vi "MultiAxisControl.vi"() -> ()   [LabVIEW 2010]
uses:
  Utility/AxisControl.ctl
  Motion/AbortSingle.vi
  Motion/MoveIncSingle.vi
  Motion/FreerunSingle.vi
  Motion/EnableSingle.vi
  Motion/DisableSingle.vi
  Motion/FaultAckSingle.vi
  Motion/HomeSingle.vi
  Parameters/GetAxisParameterString.vi
  Parameters/GetAxisParameterDouble.vi
panel:
  out "Status":string
  in  "StopProgram":bool caption="Stop"
  out "do stop":bool
  in  "stop":bool
  out "Error":string
  in  "Init":bool=TRUE
  in  "Abort Motion":bool
  in  "Reset Controller":bool
  in  "In Task:":i32(ring)=1 items=["Auxiliary", "T1", "T2", "T3", "T4"]
  in  "ExecuteProgram":bool caption="Execute"
  in  "Program:":path
  in  "Axes":T1[](array[typedef])
  in  "Status":string
  in  "Execute":bool
  in  "Command:":string
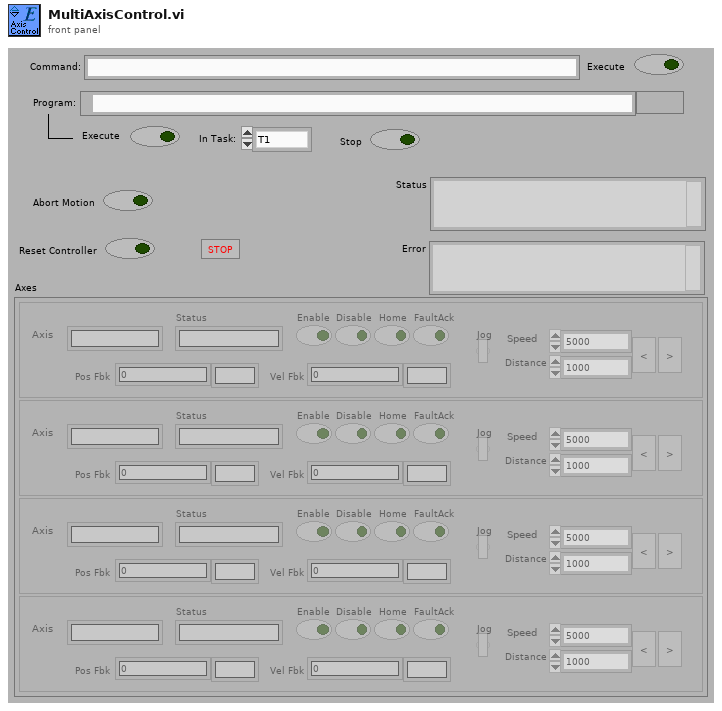
[diagram p1: front panel]
types:
  T1 = typedef "AxisControl.ctl" = cluster{"Axis":string, "Enable":bool, "Disable":bool, "Home":bool, "FaultAck":bool, "Jog":bool, "Speed":dbl, "Distance":dbl, "Jog Left":bool, "Jog Right":bool, "Status":string, "Pos Fbk":dbl, "Vel Fbk":dbl, "Pos Units":string, "Vel Units":string}
  T2 = cluster{"new reference":refnum<k24>, "Event Callback":refnum<k27>, "ControllerDiagPacket":refnum<user-event>, "Event Registration Refnum":refnum<event-registration>}
  T3 = enum32{"invalid app kind", "Development System", "Run Time System", "Student Edition", "Embedded LabVIEW", "Evaluation", "Custom"}
  T4 = cluster{"Axis":string, "Enable":bool, "Disable":bool, "Home":bool, "FaultAck":bool, "Jog":bool, "Speed":dbl, "Distance":dbl, "Jog Left":bool, "Jog Right":bool, "Status":string, "Pos Fbk":dbl, "Vel Fbk":dbl, "Pos Units":string, "Vel Units":string}
  T5 = typedef "AxisDiagPacket.ctl" = cluster{"Axis Name":string, "Acceleration Command":dbl, "Amplifier Temperature":sgl, "Analog Input 0":dbl, "Analog Input 1":dbl, "Analog Output 0":dbl, "Analog Output 1":dbl, "Axis Fault (num)":i32, "Axis Fault (str)":string, "Axis Fault (bits)":cluster{"AmplifierFault":bool, "AmplifierTemperatureFault":bool, "CcwEndOfTravelLimitFault":bool, "CcwSoftwareLimitFault":bool, "CommunicationLostFault":bool, "CwEndOfTravelLimitFault":bool, "CwSoftwareLimitFault":bool, "EmergencyStopFault":bool, "EncoderFault":bool, "ExternalFault":bool, "FeedbackScalingFault":bool, "HallSensorFault":bool, "MarkerSearchFault":bool, "MaxVelocityCommandFault":bool, "MotorTemperatureFault":bool, "None":bool, "OverCurrentFault":bool, "PositionErrorFault":bool, "PositionFeedbackFault":bool, "VelocityErrorFault":bool, "VelocityFeedbackFault":bool, "VoltageClampFault":bool, "PowerSupplyFault":bool}, "Axis Status (num)":i32, "Axis Status (str)":string, "Axis Status (bits)":cluster{"AccelerationPhase":bool, "AutofocusActive":bool, "BrakeOutput":bool, "CalibrationActive":bool, "CalibrationEnabled":bool, "CcwEndOfTravelLimitInput":bool, "CommandShapingFilterDone":bool, "CosineEncoderError":bool, "CurrentClamp":bool, "CwEndOfTravelLimitInput":bool, "DecelerationPhase":bool, "EmergencyStopInput":bool, "Enabled":bool, "GantryMasterActive":bool, "GantryModeActive":bool, "HallAInput":bool, "HallBInput":bool, "HallCInput":bool, "Homed":bool, "HomeLimitInput":bool, "Homing":bool, "InPosition":bool, "InPosition2":bool, "JoystickControl":bool, "MarkerInput":bool, "MasterMotionSuppressed":bool, "MasterSlaveControl":bool, "MotionIsCw":bool, "MoveActive":bool, "None":bool, "PositionCaptureActive":bool, "ServoControl":bool, "SineEncoderError":bool}, "Current Command":sgl, "Current Error":sgl, "Current Feedback":sgl, "Digital Input 0":i32, "Digital Input 1":i32, "Digital Input 2":i32, "Digital Output 0":i32, "Digital Output 1":i32, "Digital Output 2":i32, "Position Feedback Auxiliary":dbl, "Position Command":dbl, "Position Error":dbl, "Position Feedback":dbl, "Program Position Command":dbl, "Program Position Error":dbl, "Program Position Feedback":dbl, "Velocity Command":dbl, "Velocity Error":dbl, "Velocity Feedback":dbl}
  T6 = cluster{"Axis":string, "Enable":bool, "Disable":bool, "Home":bool, "FaultAck":bool, "Jog":bool, "Speed":dbl, "Distance":dbl, "Jog Left":bool, "Jog Right":bool, "Status":string, "Pos Fbk":dbl, "Vel Fbk":dbl, "Pos Units":string, "Vel Units":string}[]
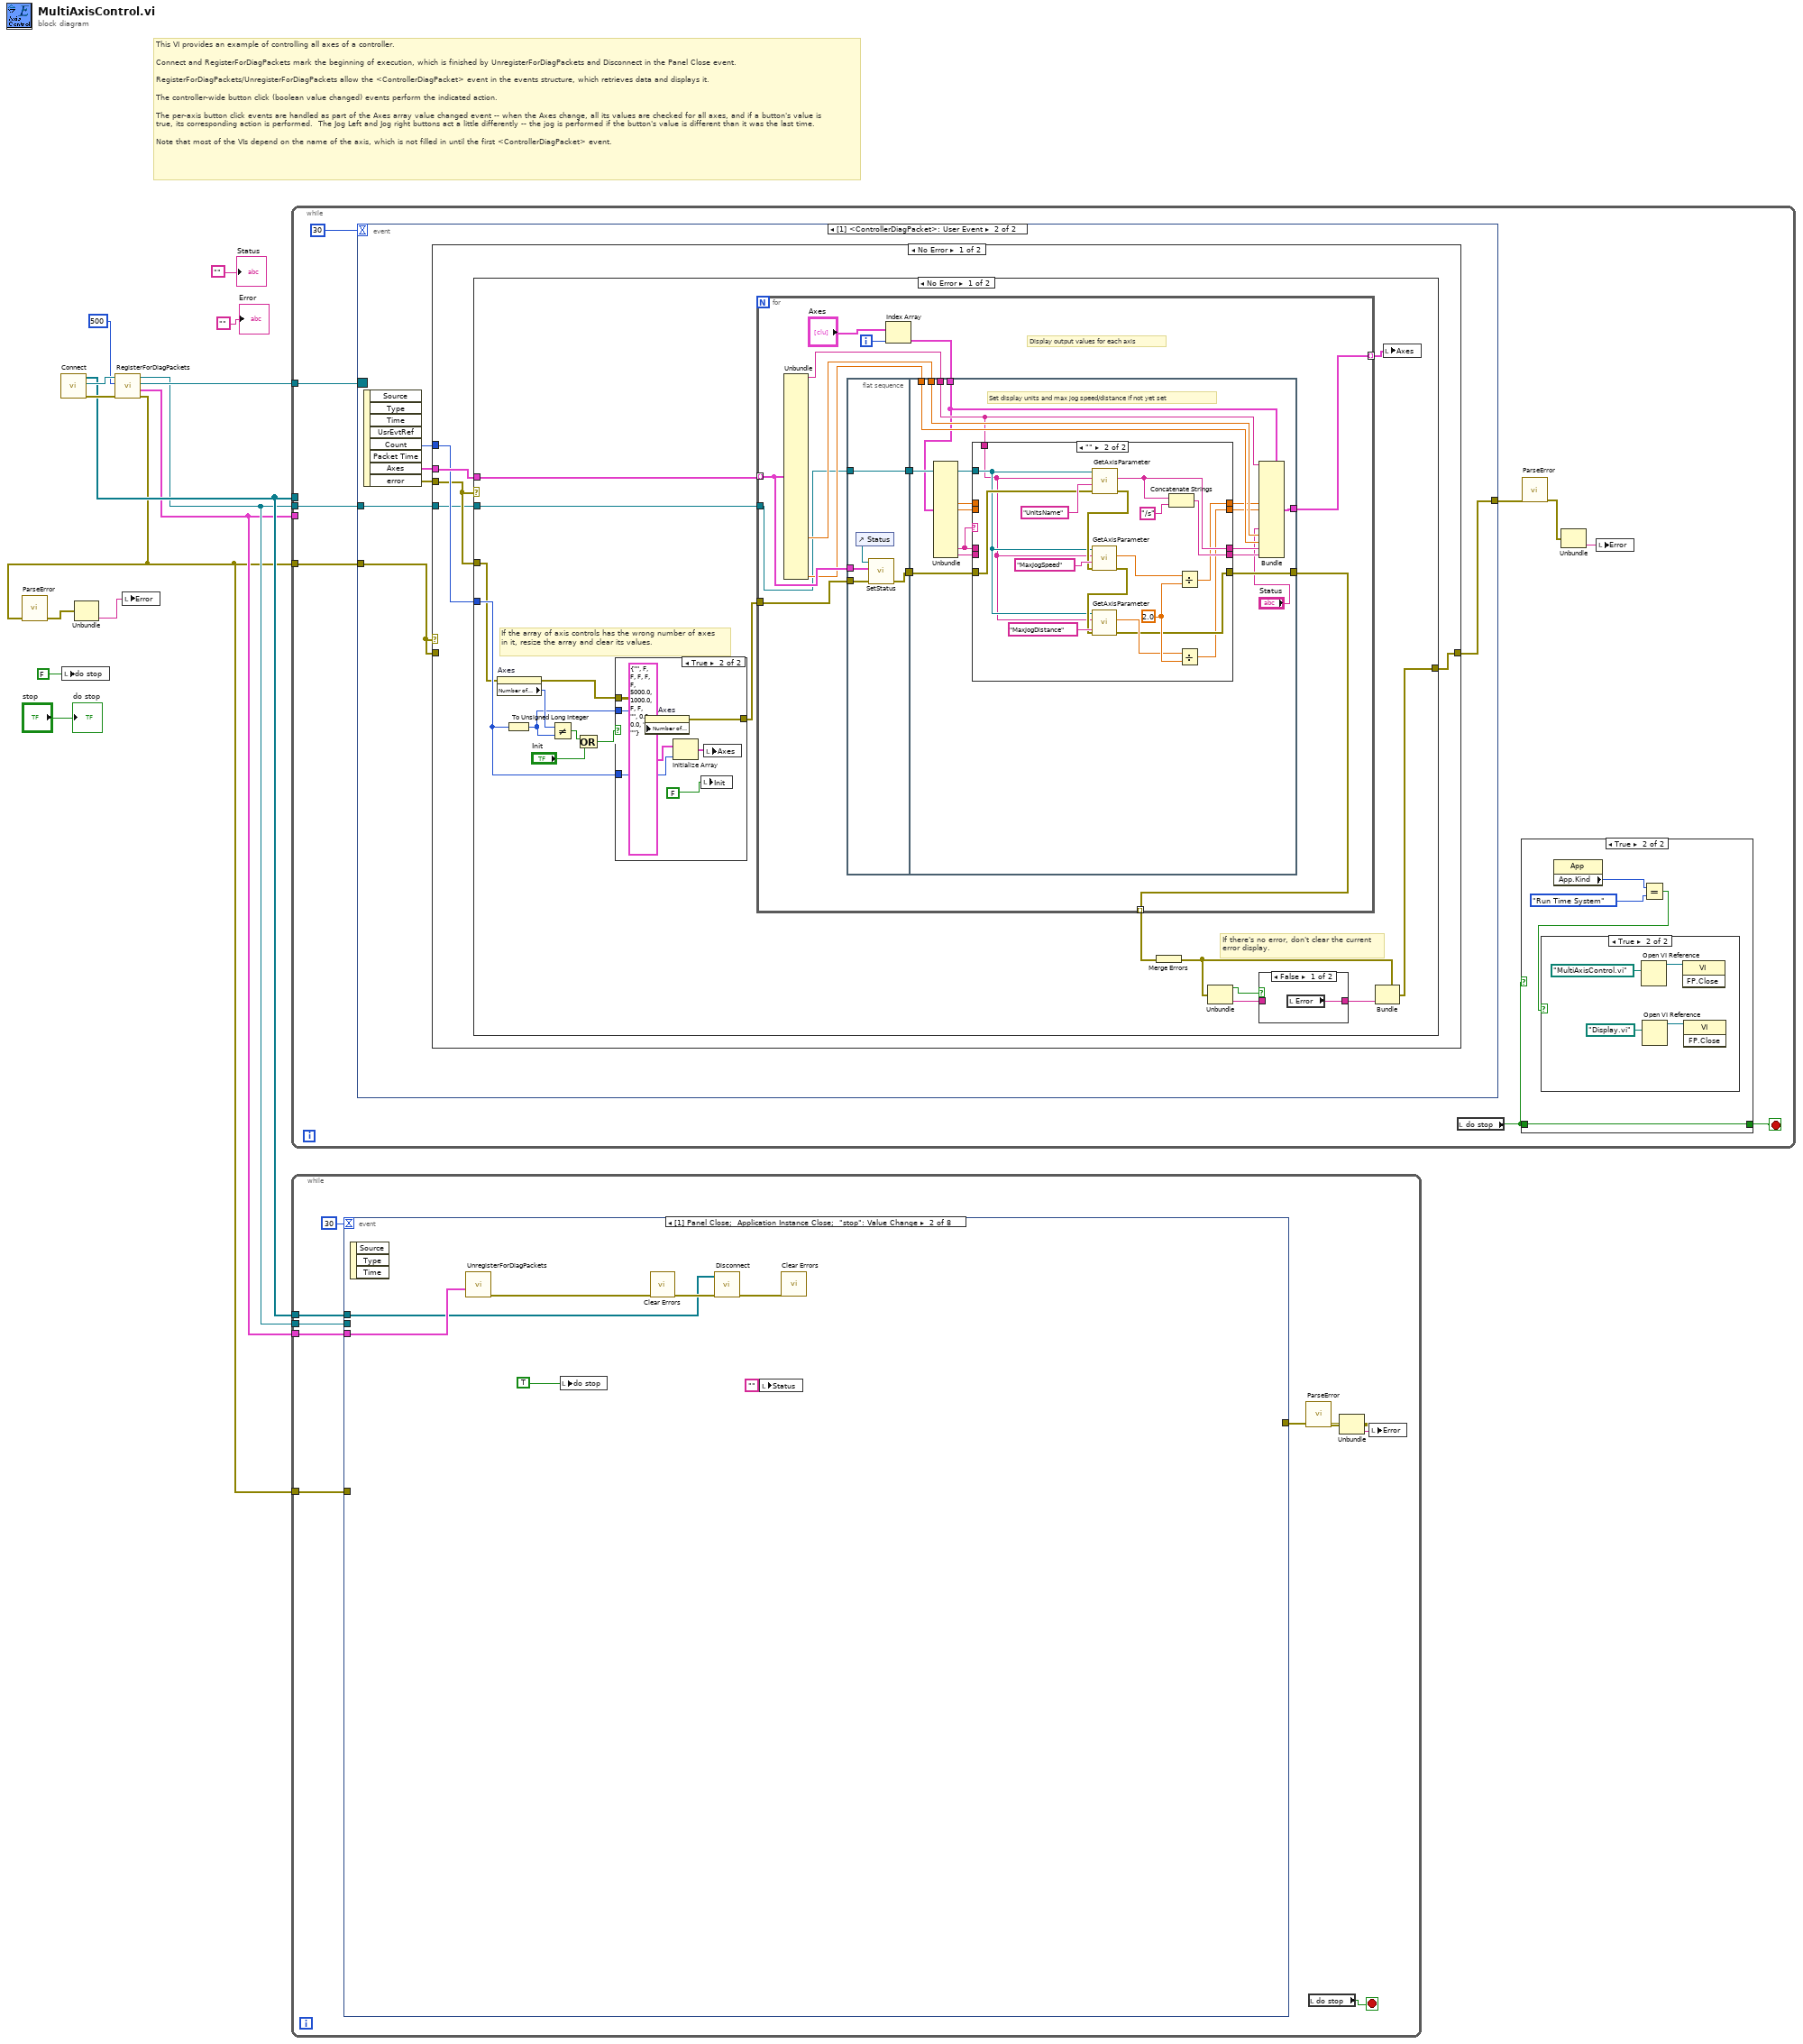
[diagram p0: block diagram]
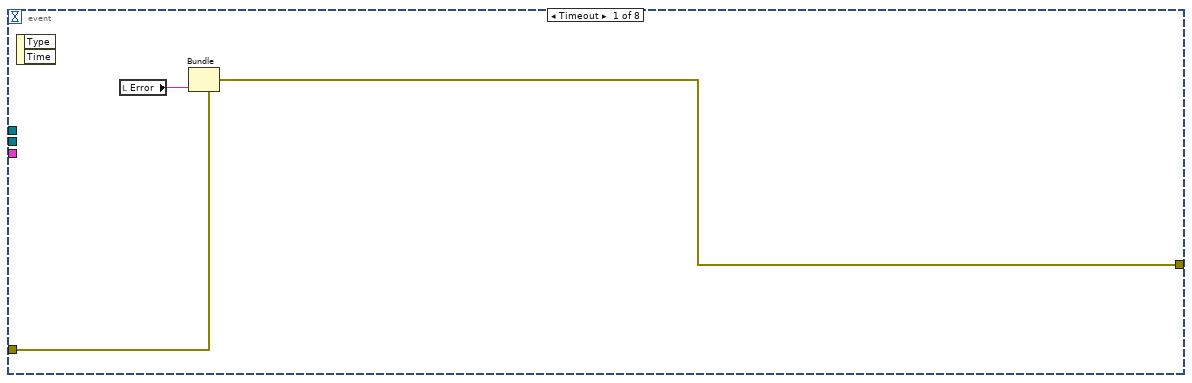
[diagram p2: hidden frame]
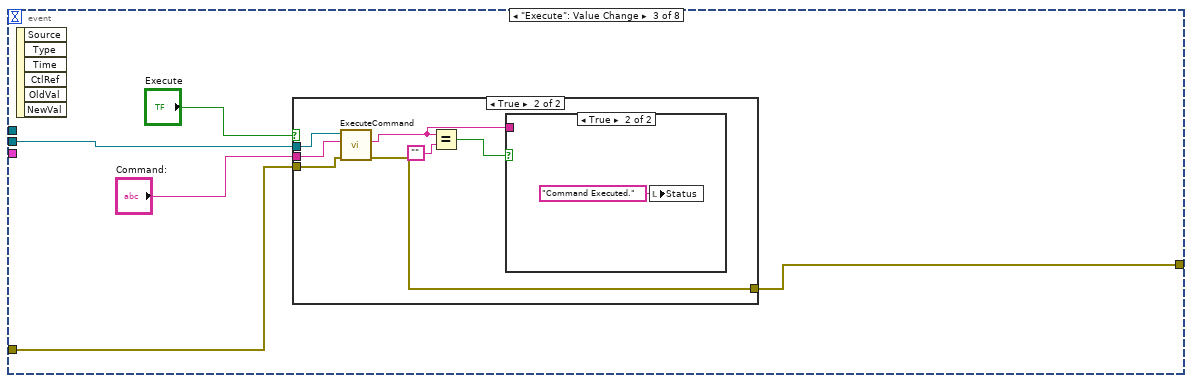
[diagram p3: hidden frame]
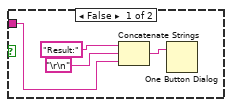
[diagram p5: hidden frame]
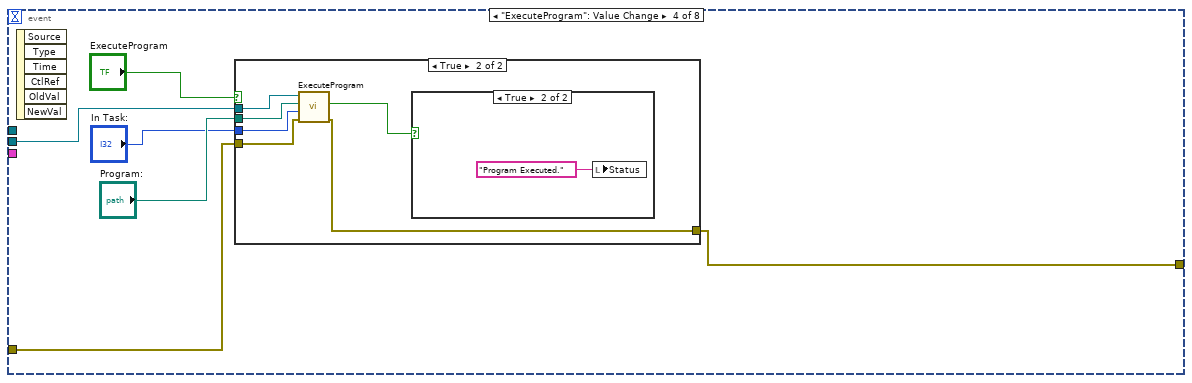
[diagram p6: hidden frame]
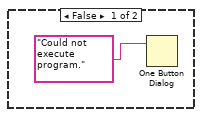
[diagram p8: hidden frame]
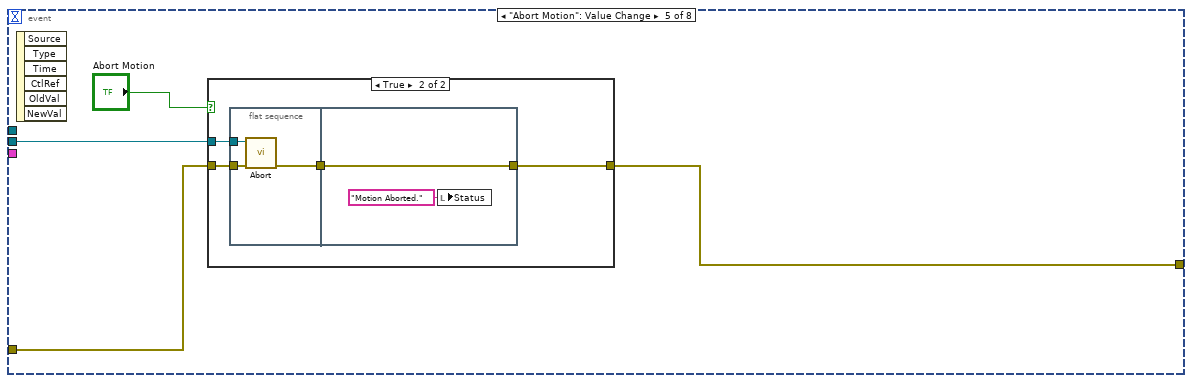
[diagram p9: hidden frame]
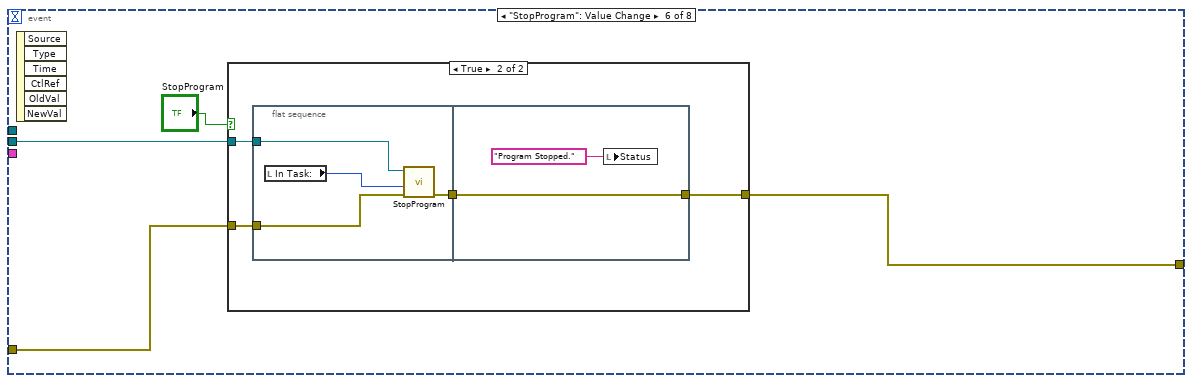
[diagram p11: hidden frame]
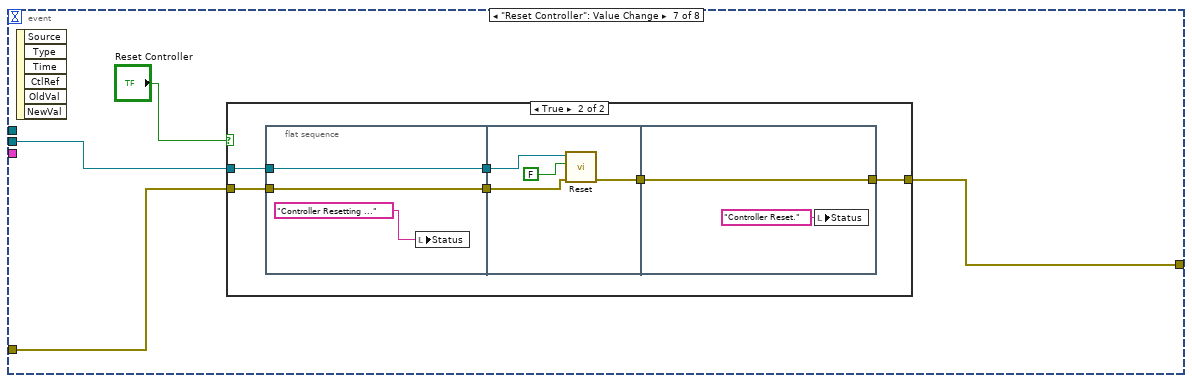
[diagram p13: hidden frame]
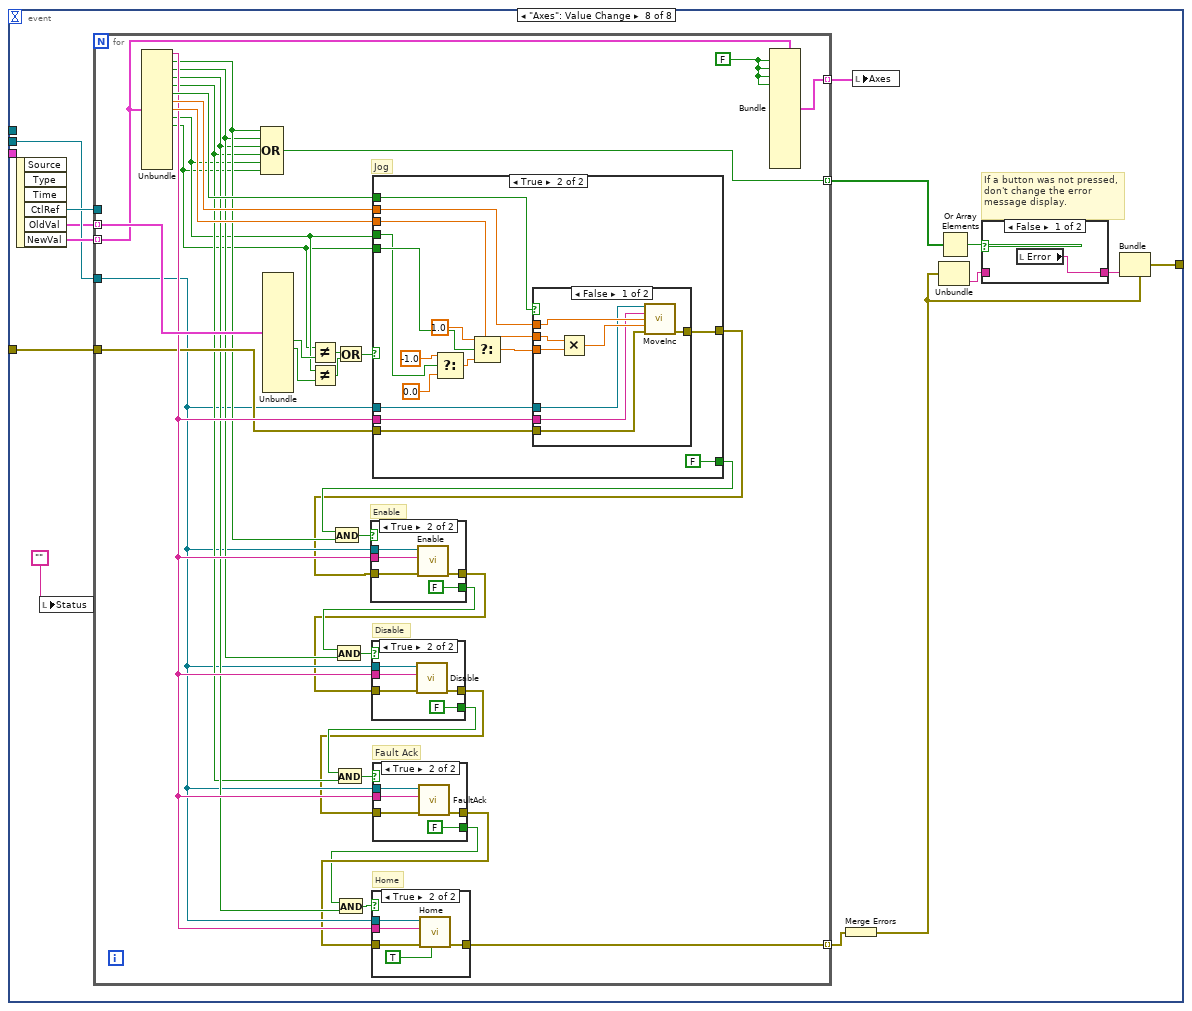
[diagram p15: hidden frame]
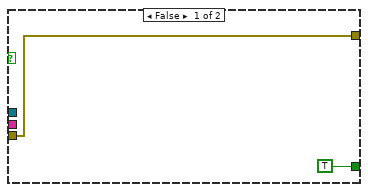
[diagram p17: hidden frame]
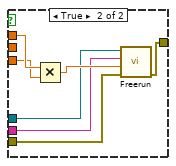
[diagram p18: hidden frame]
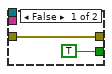
[diagram p19: hidden frame]
diagram:
  # "This VI provides an example of controlling all axes of a controller. \n\nConnect and RegisterForDiagPackets mark the beginning of execution, which is finished by UnregisterForDiagPackets and Disconnect in the Panel Close event.\n\nRegisterForDiagPackets/UnregisterForDiagPackets allow the <ControllerDiagPacket> event in the events structure, which retrieves data and displays it.\n\nThe controller-wide button click (boolean value changed) events perform the indicated action.\n\nThe per-axis button click events are handled as part of the Axes array value changed event -- when the Axes change, all its values are checked for all axes, and if a button's value is true, its corresponding action is performed.  The Jog Left and Jog right buttons act a little differently -- the jog is performed if the button's value is different than it was the last time.\n\nNote that most of the VIs depend on the name of the axis, which is not filled in until the first <ControllerDiagPacket> event."
  n1 = call "Connect.vi"() -> ("error out"=w12:errorcluster, "controller"=w13:refnum<k24>, "controllers"=w7:refnum<k24>[])  [unwired: 9 in]
  n2 = local write "do stop"(FALSE ("do stop")) -> ()
  n3 = call "RegisterForDiagPackets.vi"("error in (no error)"=w12, "refresh interval (default)"=500, "Controller in"=w13) -> ("error out"=w4:errorcluster, "Even Metadata"=w5:T2, "Event Registration Refnum"=w14:refnum<event-registration>, "Controller out"=w6:refnum<k24>)  [unwired: 4 in]
  n4 = call "ParseError.vi"("error in (no error)"=w4) -> ("error out"=w9:errorcluster)  [unwired: 10 in]
  n5 = Unbundle(w9) -> ("source"=w10:string)  [unwired: 2 out]
  n6 = local write "Error"(w10) -> ()
  n7 = while {
    tunnel: w14 -> [w20]
    tunnel: w5 -> [_]
    tunnel: w6 -> [w18]
    tunnel: w7 -> [_]
    tunnel: w4 -> [w17]
    stop <- w16 stop-if-true
    n8 = event shown="[1] <ControllerDiagPacket>: User Event" {
      selector: w20 -> [_ _]
      dyn-events: _ -> [_ _]
      timeout: 30 -> [_ _]
      tunnel: [w33 w41] -> w19
      tunnel: w18 -> [_ w40]
      tunnel: w17 -> [w35 w39]
      event Timeout {
        n9 = event-data() -> ()  [unwired: 1 in, 2 out]
        n10 = local read "Error"() -> (w34:string)
        n11 = Bundle(cluster=w35, "source"=w34) -> (w33:errorcluster)  [unwired: 2 in]
      }
      event User Event {
        n12 = event-data() -> ("Count"=w38:i32, "Axes"=w37:T5[], "error"=w36:errorcluster)  [unwired: 1 in, 5 out]
        n13 = case shown="No Error" w39 {
          tunnel: w37 -> [w46 _]
          tunnel: [w45 w133] -> w41
          tunnel: w38 -> [w44 _]
          tunnel: w36 -> [w43 _]
          tunnel: w39 -> [_ w133]
          tunnel: w40 -> [w42 _]
          frame No Error {
            n14 = case shown="No Error" w43 {
              tunnel: w46 -> [w64 _]
              tunnel: [w53 w132] -> w45
              tunnel: w43 -> [w49 w132]
              tunnel: w44 -> [w58 _]
              tunnel: w42 -> [w47 _]
              frame No Error {
                # "If there's no error, don't clear the current error display."
                # "If the array of axis controls has the wrong number of axes in it, resize the array and clear its values."
                n15 = property on="Axes" class="Arr (strict)"(error in=w49) -> (error out=w48:errorcluster, "Number of Rows"=w60:u32)  [unwired: 1 in, 1 out]
                n16 = To Unsigned Long Integer(number=w58) -> (unsigned 32bit integer=w59:u32)
                n17 = Not Equal?(x=w60, y=w59) -> (x != y?=w57:bool)
                n18 = Or(x=w57, y="Init") -> (x .or. y?=w56:bool)
                n19 = case shown="True" w56 {
                  tunnel: w48 -> [w124 w131]
                  tunnel: [w124 w130] -> w63
                  tunnel: w59 -> [_ w126]
                  tunnel: w58 -> [_ w127]
                  frame False {
                  }
                  frame True {
                    n20 = property on="Axes" class="Arr (strict)"(error in=w131, "Number of Rows"=w126) -> (error out=w130:errorcluster)  [unwired: 1 in, 1 out]
                    n21 = Initialize Array(T4 {"Axis"="", "Enable"=FALSE, "Disable"=FALSE, "Home"=FALSE, "FaultAck"=FALSE, "Jog"=FALSE, "Speed"=5000.0, "Distance"=1000.0, "Jog Left"=FALSE, "Jog Right"=FALSE, "Status"="", "Pos Fbk"=0.0, "Vel Fbk"=0.0, "Pos Units"="", "Vel Units"=""} ("Axis"), w127) -> (w129:T6)
                    n22 = local write "Init"(FALSE ("Init")) -> ()
                    n23 = local write "Axes"(w129) -> ()
                  }
                }
                n24 = for {
                  tunnel: w63 -> [w78]
                  tunnel: w64 -> [w79] mode=indexing
                  tunnel: [w77] -> w62 mode=indexing
                  tunnel: [w70] -> w61 mode=indexing
                  tunnel: w47 -> [w68]
                  i -> [w73]
                  # "Display output values for each axis"
                  n25 = Unbundle(w79) -> ("Axis Name"=w76:string, "Position Feedback"=w72:dbl, "Velocity Feedback"=w71:dbl)  [unwired: 29 out]
                  n26 = flat-sequence {
                    tunnel: w79 -> [w83]
                    tunnel: w78 -> [w82]
                    tunnel: [w81] -> w69
                    tunnel: w68 -> [w80]
                    tunnel: [w80] -> w67
                    tunnel: w74 -> [w94]
                    tunnel: w76 -> [w96]
                    tunnel: w72 -> [w100]
                    tunnel: w71 -> [w99]
                    tunnel: w69 -> [w97]
                    tunnel: w67 -> [w95]
                    tunnel: [w101] -> w77
                    tunnel: [w98] -> w70
                    frame #0 {
                      n27 = control-ref of="Status"() -> (w84:refnum<vi>)
                      n28 = call "SetStatus.vi"("error in (no error)"=w82, "AxisDiagPacket"=w83, "Status string"=w84) -> ("error out"=w81:errorcluster)  [unwired: 8 in]
                    }
                    frame #1 {
                      # "Set display units and max jog speed/distance if not yet set"
                      n29 = Unbundle(w94) -> ("Speed"=w89:dbl, "Distance"=w88:dbl, "Pos Units"=w93:string, "Vel Units"=w92:string)  [unwired: 11 out]
                      n30 = case shown="\"\"" w93 {
                        tunnel: w95 -> [_ w108]
                        tunnel: [w106 w111] -> w98
                        tunnel: w97 -> [w106 w121]
                        tunnel: w96 -> [_ w107]
                        tunnel: w93 -> [w104 _]
                        tunnel: w92 -> [w105 _]
                        tunnel: [w105 w120] -> w91
                        tunnel: [w104 w119] -> w90
                        tunnel: w89 -> [w103 _]
                        tunnel: w88 -> [w102 _]
                        tunnel: [w103 w110] -> w87
                        tunnel: [w102 w109] -> w86
                        frame Default {
                        }
                        frame "" {
                          w118 = 2.0 ("y")
                          n31 = call-poly "GetAxisParameter.vi"("error in (no error)"=w121, "Parameter Name"="UnitsName" ("parameter name"), "axis name"=w107, "controller in"=w108) -> ("error out"=w112:errorcluster, "value"=w119:string)  [unwired: 5 in, 1 out]
                          n32 = call-poly "GetAxisParameter.vi"("error in (no error)"=w112, "Parameter Name"="MaxJogSpeed" ("parameter name"), "axis name"=w107, "controller in"=w108) -> ("error out"=w113:errorcluster, "value"=w116:dbl)  [unwired: 5 in, 1 out]
                          n33 = call-poly "GetAxisParameter.vi"("error in (no error)"=w113, "Parameter Name"="MaxJogDistance" ("parameter name"), "axis name"=w107, "controller in"=w108) -> ("error out"=w111:errorcluster, "value"=w117:dbl)  [unwired: 5 in, 1 out]
                          n34 = Concatenate Strings(w119, "/s" ("string")) -> (w120:string)
                          n35 = Divide(x=w116, y=w118) -> (x/y=w110:dbl)
                          n36 = Divide(x=w117, y=w118) -> (x/y=w109:dbl)
                        }
                      }
                      n37 = Bundle(cluster=w94, "Axis"=w96, "Speed"=w87, "Distance"=w86, "Status"="Status", "Pos Fbk"=w100, "Vel Fbk"=w99, "Pos Units"=w90, "Vel Units"=w91) -> (w101:T1)  [unwired: 7 in]
                    }
                  }
                  n38 = Index Array(array="Axes", index=w73) -> (element=w74:T1)
                }
                n39 = Merge Errors(w61) -> (w54:errorcluster)
                n40 = Unbundle(w54) -> ("status"=w52:bool, "source"=w51:string)  [unwired: 1 out]
                n41 = case shown="False" w52 {
                  tunnel: w51 -> [_ w66]
                  tunnel: [w65 w66] -> w50
                  frame False {
                    n42 = local read "Error"() -> (w65:string)
                  }
                  frame True {
                  }
                }
                n43 = Bundle(cluster=w54, "source"=w50) -> (w53:errorcluster)  [unwired: 2 in]
                n44 = local write "Axes"(w62) -> ()
              }
              frame Error {
              }
            }
          }
          frame Error {
          }
        }
      }
    }
    n45 = local read "do stop"() -> (w15:bool)
    n46 = case shown="True" w15 {
      tunnel: w15 -> [w24 w28]
      tunnel: [w24 w28] -> w16
      frame False {
      }
      frame True {
        n47 = property class="App"() -> ("App.Kind"=w27:T3)  [unwired: 2 in, 2 out]
        n48 = Equal?(x=w27, y=T3."Run Time System" ("Application:Kind")) -> (x = y?=w25:bool)
        n49 = case shown="True" w25 {
          frame False {
          }
          frame True {
            n50 = Open VI Reference(vi path=path "MultiAxisControl.vi") -> (vi reference=w32:refnum<vi>)  [unwired: 5 in, 1 out]
            n51 = Open VI Reference(vi path=path "Display.vi") -> (vi reference=w30:refnum<vi>)  [unwired: 5 in, 1 out]
            n52 = invoke class="VI" method="FP.Close"(reference=w32) -> ()  [unwired: 2 in, 3 out]
            n53 = invoke class="VI" method="FP.Close"(reference=w30) -> ()  [unwired: 2 in, 3 out]
          }
        }
      }
    }
    n54 = call "ParseError.vi"("error in (no error)"=w19) -> ("error out"=w22:errorcluster)  [unwired: 10 in]
    n55 = Unbundle(w22) -> ("source"=w23:string)  [unwired: 2 out]
    n56 = local write "Error"(w23) -> ()
  }
  n57 = while {
    tunnel: w7 -> [w138]
    tunnel: w6 -> [w137]
    tunnel: w5 -> [w136]
    tunnel: w4 -> [w135]
    stop <- w134 stop-if-true
    n58 = event shown="[1] Panel Close;  Application Instance Close;  \"stop\": Value Change" {
      selector: _ -> [_ _ _ _ _ _ _ _]
      dyn-events: _ -> [_ _ _ _ _ _ _ _]
      timeout: 30 -> [_ _ _ _ _ _ _ _]
      tunnel: w136 -> [_ w152 _ _ _ _ _ _]
      tunnel: w137 -> [_ _ w156 w175 w188 w200 w217 w246]
      tunnel: w135 -> [w145 _ w155 w173 w189 w202 w216 w245]
      tunnel: [w144 _ w153 w171 w186 w201 w215 w240] -> w140
      tunnel: w138 -> [_ w149 _ _ _ _ _ _]
      event Timeout {
        n59 = event-data() -> ()  [unwired: 1 in, 2 out]
        n60 = local read "Error"() -> (w143:string)
        n61 = Bundle(cluster=w145, "source"=w143) -> (w144:errorcluster)  [unwired: 2 in]
      }
      event Panel Close; Application Instance Close; "stop": Value Change {
        n62 = event-data() -> ()  [unwired: 1 in, 3 out]
        n63 = call "UnregisterForDiagPackets.vi"("Even Metadata"=w152) -> ("error out"=w151:errorcluster)  [unwired: 10 in]
        n64 = local write "do stop"(TRUE) -> ()
        n65 = call <vilib>:"Clear Errors.vi"("error in (no error)"=w151) -> ("error out"=w150:errorcluster)  [unwired: 6 in]
        n66 = call "Disconnect.vi"("error in (no error)"=w150, "controllers"=w149) -> ("error out"=w148:errorcluster)  [unwired: 9 in]
        n67 = local write "Status"("") -> ()
        n68 = call <vilib>:"Clear Errors.vi"("error in (no error)"=w148) -> ()  [unwired: 6 in, 1 out]
      }
      event "Execute": Value Change {
        n69 = event-data() -> ()  [unwired: 1 in, 6 out]
        n70 = case shown="True" "Execute" {
          tunnel: w156 -> [_ w165]
          tunnel: w155 -> [w158 w163]
          tunnel: "Command:" -> [_ w164]
          tunnel: [w158 w159] -> w153
          frame False {
          }
          frame True {
            n71 = call "ExecuteCommand.vi"("error in (no error)"=w163, "code"=w164, "controller in"=w165) -> ("error out"=w159:errorcluster, "return value"=w160:string)  [unwired: 6 in, 1 out]
            n72 = Equal?(x=w160, y="") -> (x = y?=w161:bool)
            n73 = case shown="True" w161 {
              tunnel: w160 -> [w166 _]
              frame False {
                n74 = Concatenate Strings("Result:", "\r\n", w166) -> (w169:string)
                n75 = One Button Dialog(message=w169) -> ()  [unwired: 1 in, 1 out]
              }
              frame True {
                n76 = local write "Status"("Command Executed." ("Status")) -> ()
              }
            }
          }
        }
      }
      event "ExecuteProgram": Value Change {
        n77 = event-data() -> ()  [unwired: 1 in, 6 out]
        n78 = case shown="True" "ExecuteProgram" {
          tunnel: w175 -> [_ w183]
          tunnel: w173 -> [w177 w181]
          tunnel: "Program:" -> [_ w182]
          tunnel: "In Task:" -> [_ w179]
          tunnel: [w177 w178] -> w171
          frame False {
          }
          frame True {
            n79 = call "ExecuteProgram.vi"("error in (no error)"=w181, "task id"=w179, "path"=w182, "controller in"=w183) -> ("error out"=w178:errorcluster, "success"=w180:bool)  [unwired: 5 in, 1 out]
            n80 = case shown="True" w180 {
              frame False {
                n81 = One Button Dialog(message="Could not execute program.") -> ()  [unwired: 1 in, 1 out]
              }
              frame True {
                n82 = local write "Status"("Program Executed." ("Status")) -> ()
              }
            }
          }
        }
      }
      event "Abort Motion": Value Change {
        n83 = event-data() -> ()  [unwired: 1 in, 6 out]
        n84 = case shown="True" "Abort Motion" {
          tunnel: w188 -> [_ w194]
          tunnel: w189 -> [w190 w193]
          tunnel: [w190 w192] -> w186
          frame False {
          }
          frame True {
            n85 = flat-sequence {
              tunnel: w194 -> [w197]
              tunnel: w193 -> [w196]
              tunnel: [w195] -> w191
              tunnel: [w199] -> w192
              tunnel: w191 -> [w199]
              frame #0 {
                n86 = call-poly "Abort.vi"("error in (no error)"=w196, "controller in"=w197) -> ("error out"=w195:errorcluster)  [unwired: 8 in, 1 out]
              }
              frame #1 {
                n87 = local write "Status"("Motion Aborted." ("Status")) -> ()
              }
            }
          }
        }
      }
      event "StopProgram": Value Change {
        n88 = event-data() -> ()  [unwired: 1 in, 6 out]
        n89 = case shown="True" "StopProgram" {
          tunnel: w202 -> [w204 w208]
          tunnel: [w204 w207] -> w201
          tunnel: w200 -> [_ w206]
          frame False {
          }
          frame True {
            n90 = flat-sequence {
              tunnel: w208 -> [w211]
              tunnel: w206 -> [w209]
              tunnel: [w210] -> w205
              tunnel: [w214] -> w207
              tunnel: w205 -> [w214]
              frame #0 {
                n91 = local read "In Task:"() -> (w212:i32)
                n92 = call "StopProgram.vi"("error in (no error)"=w211, "task id"=w212, "controller in"=w209) -> ("error out"=w210:errorcluster)  [unwired: 7 in, 1 out]
              }
              frame #1 {
                n93 = local write "Status"("Program Stopped." ("Status")) -> ()
              }
            }
          }
        }
      }
      event "Reset Controller": Value Change {
        n94 = event-data() -> ()  [unwired: 1 in, 6 out]
        n95 = case shown="True" "Reset Controller" {
          tunnel: w217 -> [_ w225]
          tunnel: w216 -> [w219 w224]
          tunnel: [w219 w223] -> w215
          frame False {
          }
          frame True {
            n96 = flat-sequence {
              tunnel: w224 -> [w227]
              tunnel: w225 -> [w228]
              tunnel: [w228] -> w222
              tunnel: [w227] -> w221
              tunnel: w222 -> [w232]
              tunnel: w221 -> [w231]
              tunnel: [w229] -> w220
              tunnel: [w234] -> w223
              tunnel: w220 -> [w234]
              frame #0 {
                n97 = local write "Status"("Controller Resetting ..." ("Errors")) -> ()
              }
              frame #1 {
                n98 = call "Reset.vi"("error in (no error)"=w231, "restart programs? (false)"=FALSE ("restartPrograms"), "controller in"=w232) -> ("error out"=w229:errorcluster)  [unwired: 7 in, 1 out]
              }
              frame #2 {
                n99 = local write "Status"("Controller Reset." ("Status")) -> ()
              }
            }
          }
        }
      }
      event "Axes": Value Change {
        # "If a button was not pressed, don't change the error message display."
        n100 = event-data() -> ("CtlRef"=w247:refnum<vi>, "OldVal"=w244:T1[], "NewVal"=w248:T1[])  [unwired: 1 in, 3 out]
        n101 = local write "Status"("") -> ()
        n102 = for {
          tunnel: w248 -> [w269] mode=indexing
          tunnel: w247 -> [_]
          tunnel: w246 -> [w267]
          tunnel: w245 -> [w275]
          tunnel: w244 -> [w282] mode=indexing
          tunnel: [w256] -> w243 mode=indexing
          tunnel: [w252] -> w242 mode=indexing
          tunnel: [w270] -> w237 mode=indexing
          w251 = FALSE
          # "Jog"
          # "Fault Ack"
          # "Home"
          # "Disable"
          # "Enable"
          n103 = Unbundle(w269) -> ("Axis"=w276:string, "Enable"=w274:bool, "Disable"=w273:bool, "Home"=w272:bool, "FaultAck"=w271:bool, "Jog"=w283:bool, "Speed"=w285:dbl, "Distance"=w284:dbl, "Jog Left"=w268:bool, "Jog Right"=w257:bool)  [unwired: 5 out]
          n104 = Compound Arithmetic op=OR(w274, w273, w272, w271, w268, w257) -> (w252:bool)
          n105 = Unbundle(w282) -> ("Jog Left"=w278:bool, "Jog Right"=w277:bool)  [unwired: 13 out]
          n106 = Not Equal?(x=w257, y=w278) -> (x != y?=w280:bool)
          n107 = Not Equal?(x=w268, y=w277) -> (x != y?=w279:bool)
          n108 = Or(x=w280, y=w279) -> (x .or. y?=w281:bool)
          n109 = case shown="True" w281 {
            tunnel: w283 -> [_ w297]
            tunnel: w285 -> [_ w295]
            tunnel: w284 -> [_ w296]
            tunnel: w257 -> [_ w291]
            tunnel: w268 -> [_ w290]
            tunnel: w267 -> [_ w294]
            tunnel: w276 -> [_ w293]
            tunnel: w275 -> [w287 w292]
            tunnel: [w287 w289] -> w260
            tunnel: [TRUE FALSE] -> w265
            frame False {
            }
            frame True {
              n110 = Select(t=-1.0, s=w290, f=0.0) -> (s? t:f=w302:dbl)
              n111 = Select(t=1.0, s=w291, f=w302) -> (s? t:f=w298:dbl)
              n112 = case shown="False" w297 {
                tunnel: w295 -> [w305 w317]
                tunnel: w296 -> [w310 _]
                tunnel: w298 -> [w309 w316]
                tunnel: w292 -> [w308 w315]
                tunnel: w293 -> [w304 w313]
                tunnel: w294 -> [w303 w312]
                tunnel: [w307 w311] -> w289
                frame False {
                  n113 = Multiply(x=w310, y=w309) -> (x*y=w306:dbl)
                  n114 = call-poly "MoveInc.vi"("controller in"=w303, "axis name"=w304, "speed"=w305, "distance"=w306, "error in (no error)"=w308) -> ("error out"=w307:errorcluster)  [unwired: 9 in, 1 out]
                }
                frame True {
                  n115 = Multiply(x=w317, y=w316) -> (x*y=w314:dbl)
                  n116 = call-poly "Freerun.vi"("error in (no error)"=w315, "speed"=w314, "axis name"=w313, "controller in"=w312) -> ("error out"=w311:errorcluster)  [unwired: 6 in, 1 out]
                }
              }
            }
          }
          n117 = And(x=w265, y=w274) -> (x .and. y?=w266:bool)
          n118 = case shown="True" w266 {
            tunnel: w267 -> [_ w344]
            tunnel: w260 -> [w339 w343]
            tunnel: w276 -> [_ w341]
            tunnel: [w339 w342] -> w259
            tunnel: [TRUE FALSE] -> w263
            frame False {
            }
            frame True {
              n119 = call-poly "Enable.vi"("error in (no error)"=w343, "axis name"=w341, "controller in"=w344) -> ("error out"=w342:errorcluster)  [unwired: 7 in, 1 out]
            }
          }
          n120 = And(x=w263, y=w273) -> (x .and. y?=w264:bool)
          n121 = case shown="True" w264 {
            tunnel: w267 -> [_ w337]
            tunnel: w259 -> [w332 w335]
            tunnel: w276 -> [_ w336]
            tunnel: [w332 w334] -> w258
            tunnel: [TRUE FALSE] -> w261
            frame False {
            }
            frame True {
              n122 = call-poly "Disable.vi"("error in (no error)"=w335, "axis name"=w336, "controller in"=w337) -> ("error out"=w334:errorcluster)  [unwired: 7 in, 1 out]
            }
          }
          n123 = And(x=w261, y=w271) -> (x .and. y?=w262:bool)
          n124 = case shown="True" w262 {
            tunnel: w267 -> [_ w324]
            tunnel: w258 -> [w319 w322]
            tunnel: w276 -> [_ w323]
            tunnel: [w319 w321] -> w255
            tunnel: [TRUE FALSE] -> w253
            frame False {
            }
            frame True {
              n125 = call-poly "FaultAck.vi"("error in (no error)"=w322, "axis name"=w323, "controller in"=w324) -> ("error out"=w321:errorcluster)  [unwired: 7 in, 1 out]
            }
          }
          n126 = And(x=w253, y=w272) -> (x .and. y?=w254:bool)
          n127 = case shown="True" w254 {
            tunnel: w267 -> [_ w330]
            tunnel: w276 -> [_ w329]
            tunnel: w255 -> [w325 w328]
            tunnel: [w325 w327] -> w256
            frame False {
            }
            frame True {
              n128 = call-poly "Home.vi"("return immediately"=TRUE ("Return Immediately ?"), "error in (no error)"=w328, "axis name"=w329, "controller in"=w330) -> ("error out"=w327:errorcluster)  [unwired: 6 in, 1 out]
            }
          }
          n129 = Bundle(cluster=w269, "Enable"=w251, "Disable"=w251, "Home"=w251, "FaultAck"=w251) -> (w270:T1)  [unwired: 11 in]
        }
        n130 = Merge Errors(w243) -> (w236:errorcluster)
        n131 = local write "Axes"(w237) -> ()
        n132 = Unbundle(w236) -> ("source"=w239:string)  [unwired: 2 out]
        n133 = Or Array Elements(Boolean array=w242) -> (logical OR=w241:bool)
        n134 = case shown="False" w241 {
          tunnel: w239 -> [_ w250]
          tunnel: [w249 w250] -> w238
          frame False {
            n135 = local read "Error"() -> (w249:string)
          }
          frame True {
          }
        }
        n136 = Bundle(cluster=w236, "source"=w238) -> (w240:errorcluster)  [unwired: 2 in]
      }
    }
    n137 = call "ParseError.vi"("error in (no error)"=w140) -> ("error out"=w142:errorcluster)  [unwired: 10 in]
    n138 = local read "do stop"() -> (w134:bool)
    n139 = Unbundle(w142) -> ("source"=w141:string)  [unwired: 2 out]
    n140 = local write "Error"(w141) -> ()
  }
  "Error" <- ""
  "do stop" <- "stop"
  "Status" <- ""
